vi "PhotonPoseEstimator_AddHeadingData_Rotation2d.vi"(9 "Heading":T1={"VALUE"=0.0, "COS"=1.0, "SIN"=0.0} {"SIN" format="%13.4f"; "COS" format="%13.4f"; "VALUE" format="%13.4f"}, 11 "TimeStamp":dbl=-1.0) -> ()   [LabVIEW 2019, in "PhotonVisionLib.lvlib"]
doc: "Add heading data\n\nInputs: \n -- TimeStamp -- double -- System elapsed time from FPGA\n -- Heading -- Rotation2d -- Heading value\n\nOutputs:\n - none -"
uses:
  PhotonVisionLib.lvlib
  <vilib>/Rock Robotics/WPI/ThirdParty/JAS_Junk/TrajLib/TypeDef/ROTATION2D.ctl
  <vilib>/Rock Robotics/WPI/ThirdParty/JAS_Junk/TrajLib/VI/TimeInterpRotation2d_CleanUp.vi
  PhotonVision_Globals.vi
  <vilib>/gmath/interp.llb/Search Ordered Table.vi
  <vilib>/Rock Robotics/WPI/ThirdParty/JAS_Junk/TrajLib/Trajectory_Library.lvlib
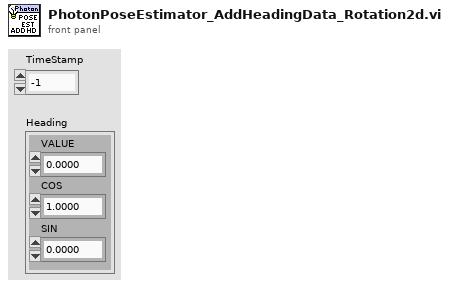
[diagram p1: front panel]
types:
  T1 = typedef "Trajectory_Library.lvlib/ROTATION2D.ctl" = cluster{"VALUE":dbl, "COS":dbl, "SIN":dbl}
  T2 = typedef "Trajectory_Library.lvlib/TIME_INTERPOLATABLE_ROTATION2D.ctl" = cluster{"TimeStamps":dbl[], "RotationValues":T1[], "Min_TimeStamp":dbl, "Max_TimeStamp":dbl, "ItemCount":i32, "MaxBufferTime":dbl}
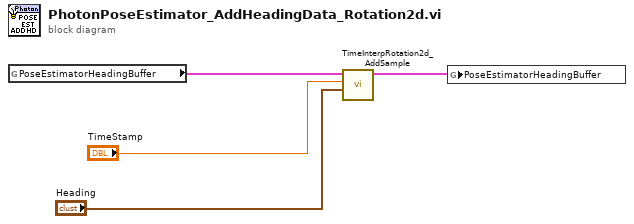
[diagram p0: block diagram]
diagram:
  n1 = global read "PhotonVision_Globals.vi" "PoseEstimatorHeadingBuffer"() -> (w1:T2)
  n2 = call <vilib>:"TimeInterpRotation2d_AddSample.vi"("RotationValue"="Heading", "TimeStamp"="TimeStamp", "in TimeInterpRotation"=w1) -> ("out TimeInterpRotation"=w4:T2)  [unwired: 7 in, 1 out]
  n3 = global write "PhotonVision_Globals.vi" "PoseEstimatorHeadingBuffer"(w4) -> ()
